vi "Get Service Interface.vi"(8 "error in":errorcluster, 11 "measurement service v2 in":refnum<class "Measurement Service V2.lvclass">) -> (0 "error out":errorcluster, 2 "service interface":string, 3 "measurement service v2 out":refnum<class "Measurement Service V2.lvclass">)   [LabVIEW 2020, in "NI Measurement Plug-In SDK.lvlib" / "Measurement Service V2.lvclass"]
uses:
  Measurement Service V2.lvclass
  Measurement Service V2.lvclass/Measurement Service V2.ctl
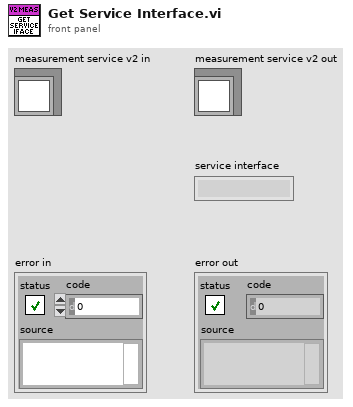
[diagram p1: front panel]
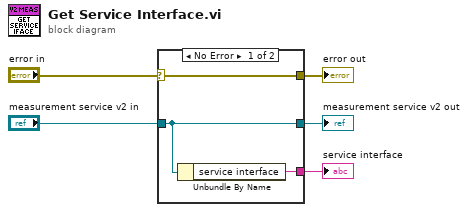
[diagram p0: block diagram]
diagram:
  n1 = case shown="No Error" "error in" {
    selector: "error in" -> [w8 w10]
    tunnel: [w8 w10] -> w4
    tunnel: [w7 w9] -> w2
    tunnel: "measurement service v2 in" -> [w7 w9]
    tunnel: [w6 _] -> w1
    frame No Error {
      n2 = Unbundle By Name(w7) -> ("service interface"=w6:string)
    }
    frame Error {
    }
  }
  "error out" <- w4
  "measurement service v2 out" <- w2
  "service interface" <- w1
